vi "WriteGain.vi"(8 "Error In":errorcluster, 10 "Gain":dbl, 11 "object in":refnum<class "Pulsetrain Config.lvclass">) -> (0 "Error Out":errorcluster, 3 "object out":refnum<class "Pulsetrain Config.lvclass">)   [LabVIEW 2023, in "Teledyne-T3AFG120.lvlib" / "Pulsetrain Config.lvclass"]
uses:
  Pulsetrain Config.lvclass
  Pulsetrain Config.lvclass/Pulsetrain Config.ctl
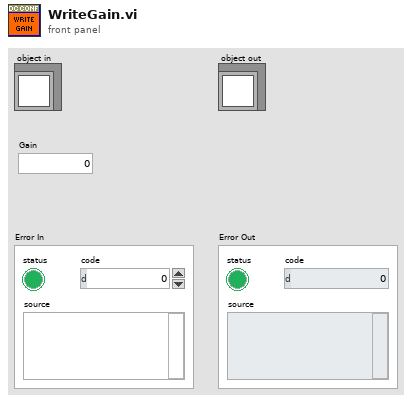
[diagram p1: front panel]
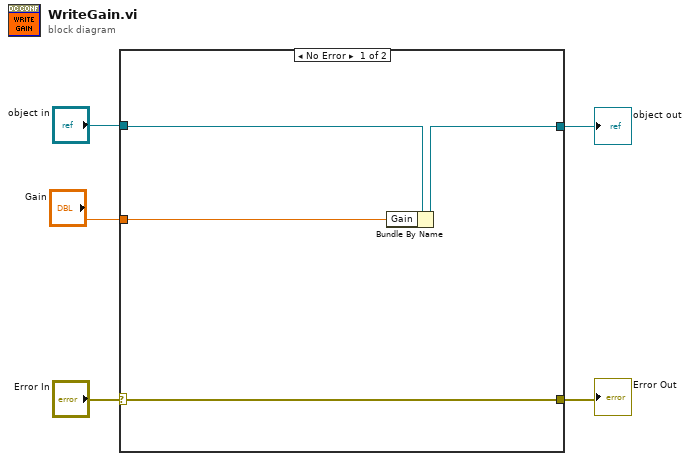
[diagram p0: block diagram]
diagram:
  n1 = case shown="No Error" "Error In" {
    selector: "Error In" -> [w8 w11]
    tunnel: [w8 w11] -> w4
    tunnel: [w6 w10] -> w2
    tunnel: "object in" -> [w7 w10]
    tunnel: "Gain" -> [w9 _]
    frame No Error {
      n2 = Bundle By Name(cluster=w7, "Gain"=w9) -> (w6:refnum<class "Pulsetrain Config.lvclass">)
    }
    frame Error {
    }
  }
  "Error Out" <- w4
  "object out" <- w2
